vi "Disque.vi"   [LabVIEW 2018]
uses:
  MyGlobal.vi
types:
  T1 = typedef "WPI_DigitalOutputDevRef.ctl" = cluster{"DIO Channel":T2, "DevStatus":errorcluster}
  T2 = typedef "FPGA_DIOChannel.ctl" = enum8{"DIO 0", "DIO 1", "DIO 2", "DIO 3", "DIO 4", "DIO 5", "DIO 6", "DIO 7", "DIO 8", "DIO 9", "DIO MXP 0", "DIO MXP 1", "DIO MXP 2", "DIO MXP 3", "DIO MXP 4", "DIO MXP 5", "DIO MXP 6", "DIO MXP 7", "DIO MXP 8", "DIO MXP 9", "DIO MXP 10", "DIO MXP 11", "DIO MXP 12", "DIO MXP 13", "DIO MXP 14", "DIO MXP 15", "SPI Port CS1", "SPI Port CS2", "SPI Port CS3", "SPI Port MISO", "SPI Port MOSI", "Invalid"}
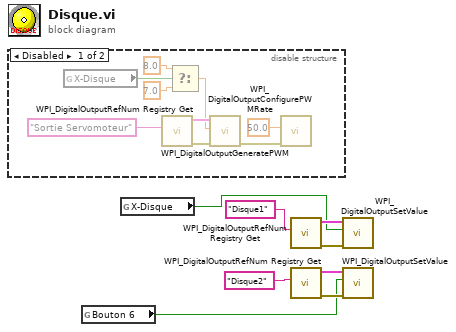
[diagram p0: block diagram]
diagram:
  n1 = disable-structure shown="Disabled" {
    frame Disabled {
      n2 = global read "MyGlobal.vi" "X-Disque"() -> (w12:bool)
      n3 = call <vilib>:"WPI_DigitalOutputRefNum Registry Get.vi"("refnum name"="Sortie Servomoteur") -> ("error out"=w15:errorcluster, "DigitalOutputDevRef"=w16:T1)  [unwired: 9 in]
      n4 = Select(t=sgl 8.0 ("PWM Duty Cycle"), s=w12, f=sgl 7.0 ("PWM Duty Cycle")) -> (s? t:f=w9:sgl)
      n5 = call <vilib>:"WPI_DigitalOutputGeneratePWM.vi"("error in (no error)"=w15, "PWM Duty Cycle"=w9, "DigitalOutputDevRef"=w16) -> ("error out"=w17:errorcluster)  [unwired: 7 in, 1 out]
      n6 = call <vilib>:"WPI_DigitalOutputConfigurePWMRate.vi"("error in (no error)"=w17, "PWM Rate (Hz)"=sgl 50.0) -> ()  [unwired: 8 in, 2 out]
    }
    frame Enabled {
    }
  }
  n7 = global read "MyGlobal.vi" "Bouton 6"() -> (w1:bool)
  n8 = global read "MyGlobal.vi" "X-Disque"() -> (w2:bool)
  n9 = call <vilib>:"WPI_DigitalOutputRefNum Registry Get.vi"("refnum name"="Disque1") -> ("error out"=w8:errorcluster, "DigitalOutputDevRef"=w7:T1)  [unwired: 9 in]
  n10 = call <vilib>:"WPI_DigitalOutputRefNum Registry Get.vi"("refnum name"="Disque2") -> ("error out"=w5:errorcluster, "DigitalOutputDevRef"=w6:T1)  [unwired: 9 in]
  n11 = call <vilib>:"WPI_DigitalOutputSetValue.vi"("error in (no error)"=w8, "Value"=w2, "DigitalOutputDevRef"=w7) -> ()  [unwired: 7 in, 2 out]
  n12 = call <vilib>:"WPI_DigitalOutputSetValue.vi"("error in (no error)"=w5, "Value"=w1, "DigitalOutputDevRef"=w6) -> ()  [unwired: 7 in, 2 out]
